vi "test Send Error Report.vi"(8 "error in (no error)":errorcluster, 11 "TestCase in":refnum<class "Test TCP Nested Endpoint Nonforwarded Messages.lvclass">) -> (0 "error out":errorcluster, 3 "TestCase out":refnum<class "Test TCP Nested Endpoint Nonforwarded Messages.lvclass">)   [LabVIEW 2020, in "Test TCP Nested Endpoint Nonforwarded Messages.lvclass"]
uses:
  Test TCP Nested Endpoint Nonforwarded Messages.lvclass
  <vilib>/addons/_JKI Toolkits/VI Tester/TestCase.llb/TestCase.lvclass
  <vilib>/ActorFramework/Message Queue/Message Queue.lvclass
  <vilib>/ActorFramework/Message Dequeuer/Message Dequeuer.lvclass
  <vilib>/ActorFramework/Report Error Msg/Report Error Msg.lvclass
  <vilib>/ActorFramework/LastAck/Last Ack.lvclass
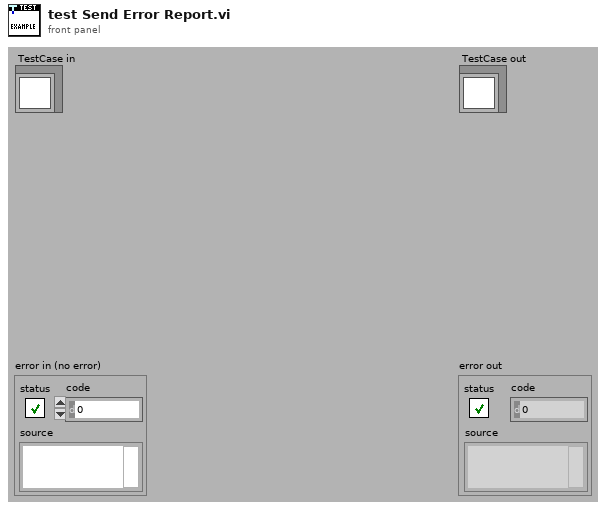
[diagram p1: front panel]
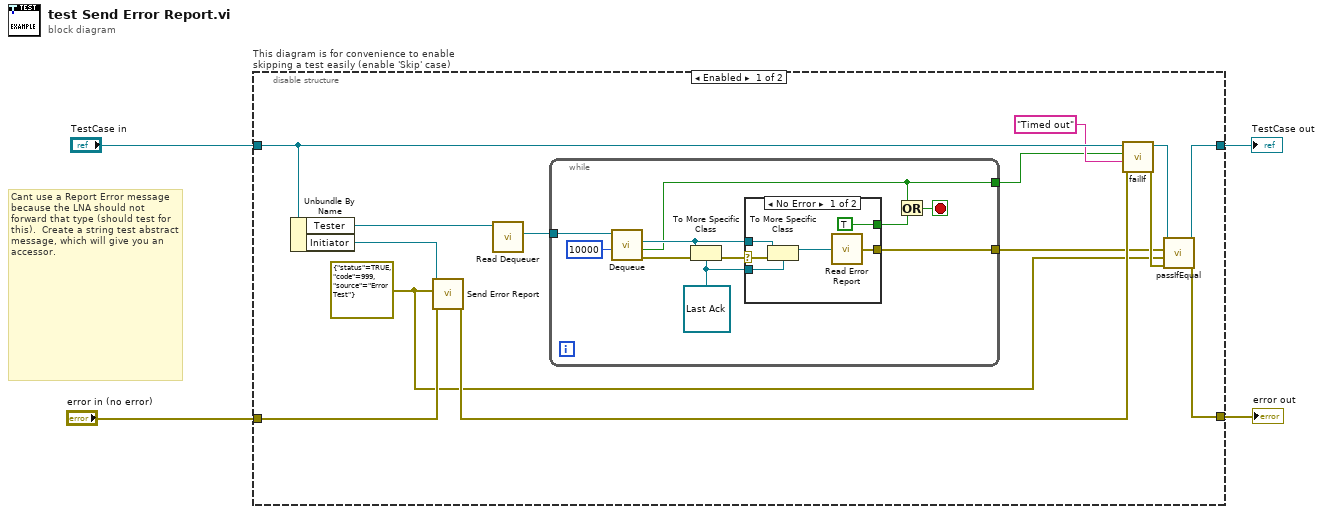
[diagram p0: block diagram]
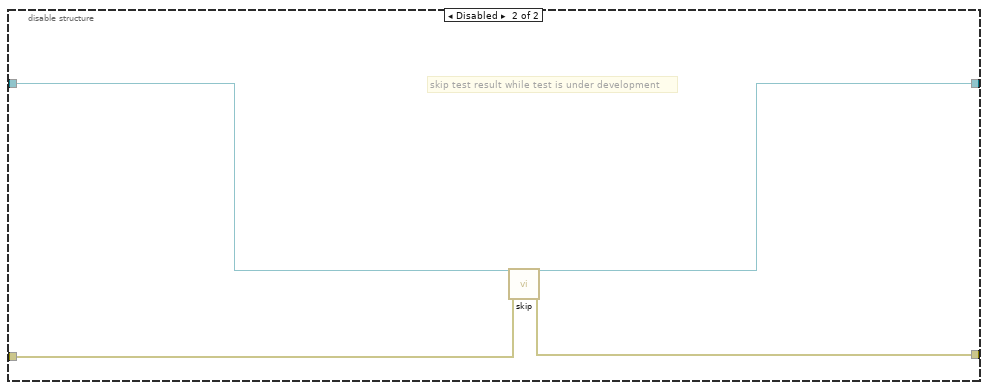
[diagram p3: hidden frame]
diagram:
  # "Cant use a Report Error message because the LNA should not forward that type (should test for this).  Create a string test abstract message, which will give you an accessor."
  n1 = disable-structure "This diagram is for convenience to enable skipping a test easily (enable 'Skip' case)" shown="Enabled" {
    disable-tunnel: "TestCase in" -> [w14 w38]
    disable-tunnel: [w18 w36] -> w1
    disable-tunnel: [w17 w37] -> w3
    disable-tunnel: "error in (no error)" -> [w9 w35]
    frame Enabled {
      w5 = errorcluster {"status"=TRUE, "code"=999, "source"="Error Test"} ("Error From Sender")
      n2 = Unbundle By Name(w14) -> ("Tester"=w15:refnum<class "Message Queue.lvclass">, "Initiator"=w10:refnum<class "Message Enqueuer.lvclass">)
      n3 = call <vilib>:"Send Error Report.vi"("error in (no error)"=w9, "Error From Sender"=w5, "Message Enqueuer"=w10) -> ("error out"=w8:errorcluster)  [unwired: 8 in]
      n4 = call <vilib>:"Read Dequeuer.vi"("Message Queue"=w15) -> ("Message Dequeuer"=w16:refnum<class "Message Dequeuer.lvclass">)  [unwired: 10 in]
      n5 = while {
        tunnel: w16 -> [w28]
        tunnel: [w21] -> w6
        tunnel: [w22] -> w7
        stop <- w19 stop-if-true
        w23 = refnum<class "Last Ack.lvclass"> refnum ("Last Ack")
        n6 = call <vilib>:"Dequeue.vi"("timeout in ms (-1)"=10000, "Message Dequeuer in"=w28) -> ("error out"=w26:errorcluster, "timed out?"=w22:bool, "Message"=w24:refnum<class "Message.lvclass">)  [unwired: 5 in, 2 out]
        n7 = To More Specific Class(target class=w23, reference=w24, error in=w26) -> (error out=w25:errorcluster)  [unwired: 1 out]
        n8 = case shown="No Error" w25 {
          selector: w25 -> [w34 _]
          tunnel: w24 -> [w33 _]
          tunnel: w23 -> [w32 _]
          tunnel: [w30 _] -> w21
          tunnel: [TRUE _] -> w20
          frame No Error {
            n9 = To More Specific Class(target class=w32, reference=w33, error in=w34) -> (specific class reference=w31:refnum<class "Last Ack.lvclass">)  [unwired: 1 out]
            n10 = call <vilib>:"Read Error Report.vi"("Last Ack"=w31) -> ("error report"=w30:errorcluster)
          }
          frame Error {
          }
        }
        n11 = Or(x=w22, y=w20) -> (x .or. y?=w19:bool)
      }
      n12 = call-dynamic "failIf.vi"("error in (no error)"=w8, "message (\"\")"="Timed out" ("message (\"\")"), "fail"=w7, "TestCase in"=w14) -> ("error out"=w12:errorcluster, "TestCase out"=w13:refnum<class "Test TCP Nested Endpoint Nonforwarded Messages.lvclass">)  [unwired: 6 in]
      n13 = call-dynamic "passIfEqual.vi"("error in (no error)"=w12, "y"=w5, "x"=w6, "TestCase in"=w13) -> ("error out"=w17:errorcluster, "TestCase out"=w18:refnum<class "Test TCP Nested Endpoint Nonforwarded Messages.lvclass">)  [unwired: 6 in]
    }
    frame Disabled {
      # "skip test result while test is under development"
      n14 = call <vilib>:"skip.vi"("error in (no error)"=w35, "TestCase in"=w38) -> ("error out"=w37:errorcluster, "TestCase out"=w36:refnum<class "Test TCP Nested Endpoint Nonforwarded Messages.lvclass">)  [unwired: 8 in]
    }
  }
  "error out" <- w3
  "TestCase out" <- w1
